vi "flow-builder.water-dosing.vi"(7 "Proc Name":string, 8 "error in":errorcluster, 9 "Unit Index":i32, 10 "AIN Simulator (NaN)":dbl=nan, 11 "Cluster":T3 {"ORP Dosing"."MIX Limit" format="%d [s]"; "ORP Dosing"."MIX Dose" format="%d [s]"; "PH Dosing"."ACID Limit" format="%d [s]"; "PH Dosing"."BASE Limit" format="%d [s]"; "PH Dosing"."ACID Dose" format="%d [s]"; "PH Dosing"."BASE Dose" format="%d [s]"; "EC Dosing"."BETA2 Limit" format="%d [s]"; "EC Dosing"."ALFA2 Limit" format="%d [s]"; "EC Dosing"."ALFA2 Dose" format="%d [s]"; "EC Dosing"."BETA2 Dose" format="%d [s]"; "EC Dosing"."BETA1 Limit" format="%d [s]"; "EC Dosing"."ALFA1 Limit" format="%d [s]"; "EC Dosing"."ALFA1 Dose" format="%d [s]"; "EC Dosing"."BETA1 Dose" format="%d [s]"; "Main"."DailyActivityHours"."Begin Time" format="ON:    %<%H:%M>T"; "Main"."DailyActivityHours"."End Time" format="OFF:    %<%H:%M>T"; "Main"."WashTimes"."Out" format="Wash out: %d [sec]"; "Main"."WashTimes"."In" format="Wash in: %d [sec]"; "Water Dosing"."Water Limit" format="%d [s]"; "Water Dosing"."Water Dose" format="%d [s]"}) -> (0 "error out":errorcluster, 1 "Not Limited?":bool, 2 "status":string, 3 "Flow out":T1[](array[typedef]))   [LabVIEW 2024]
uses:
  controls/UiNutritionPanel.ctl
  controls/UiScheduleTimestamp.ctl
  controls/UiStepBuilder.ctl
  controls/type.step-builder.ctl
  controls/enum-ntr-io-format.ctl
  io.interface.serial.vi
  <vilib>/Utility/error.llb/Clear Errors.vi
  Polymorphics/variantCtrlIo.vi
  globals/globals-engine.vi
  util.environment.vi
  util-address-parser.vi
  util-address-builder.vi
  util.DO.ToString.vi
  Polymorphics/io.command-builder.vi
  Polymorphics/io.command-builder.DO.vi
  Polymorphics/io.command-builder.AI.vi
  Polymorphics/io.command-builder.DI.vi
  io.frame.vi
  io.visa.vi
  io.responseValidator.vi
  Polymorphics/io.command-parser.DI.vi
  Polymorphics/io.command-parser.AI.vi
  step.util.flag-matching.vi
  util.file.record.vi
panel:
  # "Water"
  # "EC"
  # "PH"
  # "ORP"
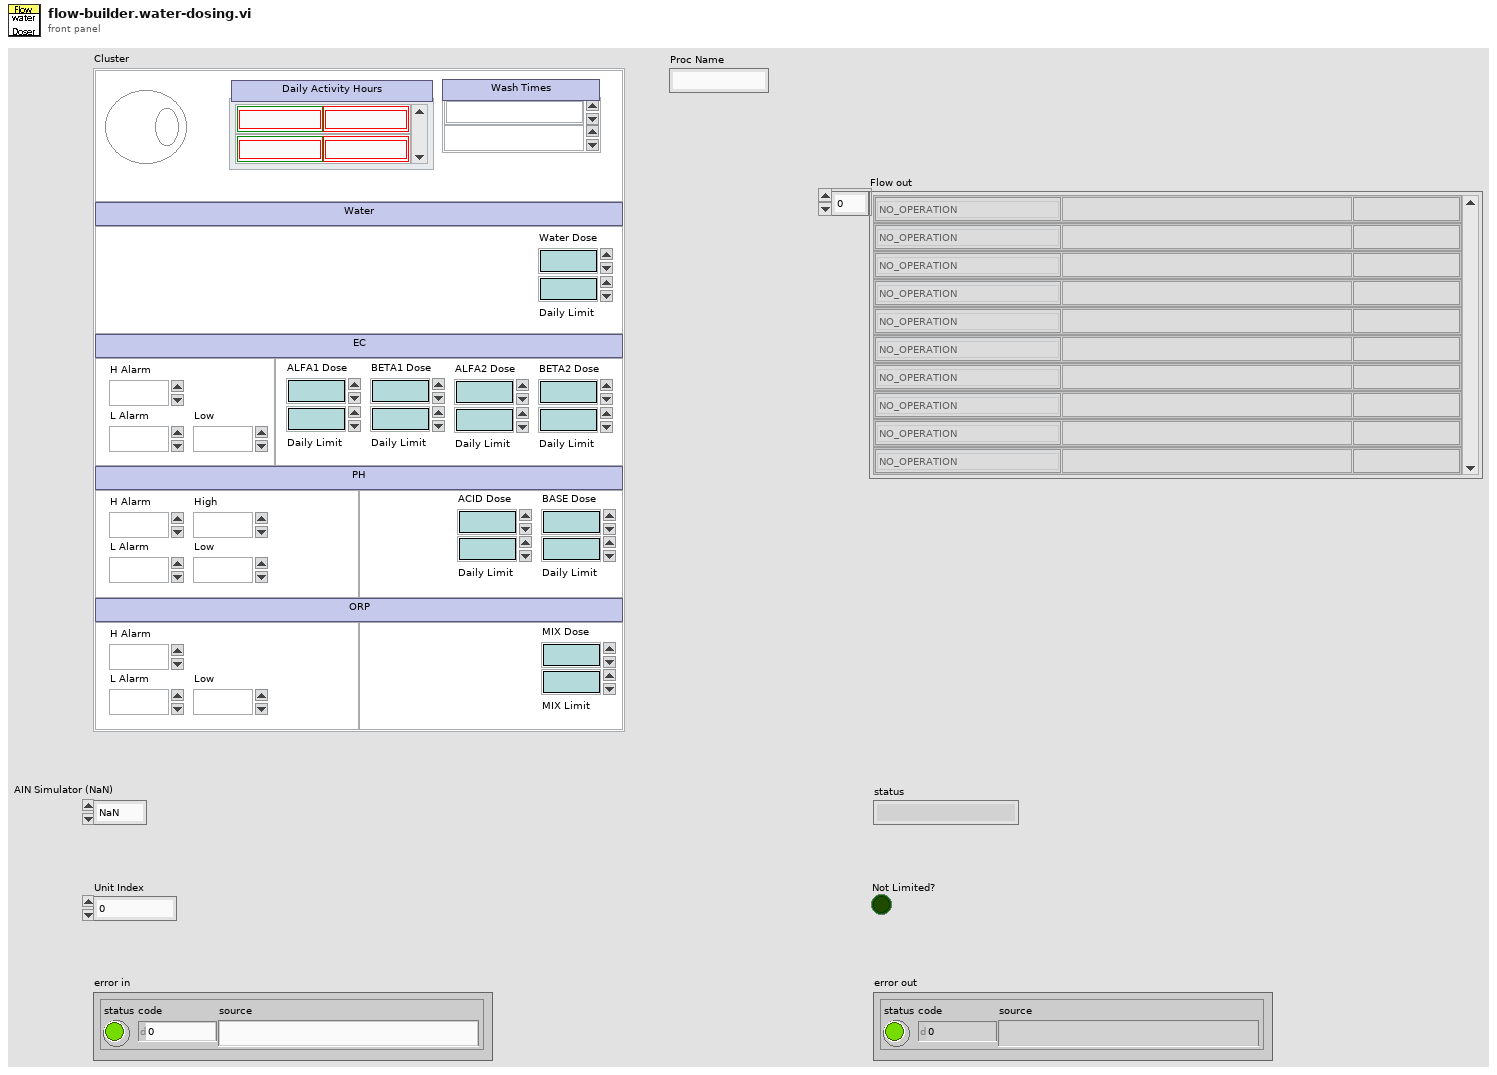
[diagram p1: front panel]
types:
  T1 = typedef "UiStepBuilder.ctl" = cluster{"Step Function":T2, "ParamString":string, "Step Label":string}
  T2 = typedef "type.step-builder.ctl" = enum16{"NO_OPERATION", "DELAY-JUMP", "DELAY", "JUMP", "COMPLETE", "SCHEDULER", "IRR-CHECK", "UNIT-CHECK", "UNIT-SAMPLE", "UNIT-DOSE", "LOG-REPORT", "LOG-MESSAGE", "IO-READ", "IO-READ-MANY", "IO-WRITE", "IO-COMPARE-OUT", "IO-COMPARE-IN", "PROC-START", "PROC-STOP", "PROC-LOAD", "PROC-IS-COMPLETED", "RECORD-MOVE", "GET-RH", "GET-UV", "GET-WD", "GET-WS", "OCS-CHECK", "OCS-RECORD"}
  T3 = typedef "UiNutritionPanel.ctl" = cluster{"Main":cluster{"Enable":bool, "WashTimes":cluster{"In":dbl, "Out":dbl}, "DailyActivityHours":cluster{"Begin Time":T4, "End Time":T4}[]}, "Water Dosing":cluster{"Water Dose":dbl, "Water Limit":dbl}, "EC Ranges":cluster{"H Alarm":dbl, "L Alarm":dbl, "Low":dbl}, "EC Dosing":cluster{"ALFA1 Dose":dbl, "ALFA1 Limit":dbl, "BETA1 Dose":dbl, "BETA1 Limit":dbl, "ALFA2 Dose":dbl, "ALFA2 Limit":dbl, "BETA2 Dose":dbl, "BETA2 Limit":dbl}, "PH Ranges":cluster{"H Alarm":dbl, "L Alarm":dbl, "High":dbl, "Low":dbl}, "PH Dosing":cluster{"ACID Dose":dbl, "ACID Limit":dbl, "BASE Dose":dbl, "BASE Limit":dbl}, "ORP Ranges":cluster{"H Alarm":dbl, "L Alarm":dbl, "Low":dbl}, "ORP Dosing":cluster{"MIX Dose":dbl, "MIX Limit":dbl}}
  T4 = typedef "UiScheduleTimestamp.ctl" = timestamp
  T5 = typedef "enum-ntr-io-format.ctl" = enum16{"UN_VLV%d", "UN_PMP%d", "UN_WL%d", "UN_PH", "UN_EC", "UN_ORP", "UN_WT", "UN_PH2", "UN_ALFA1", "UN_BETA1", "UN_ALFA2", "UN_BETA2", "UN_ACID", "UN_BASE", "UN_WATER", "UN_ORPMIX"}
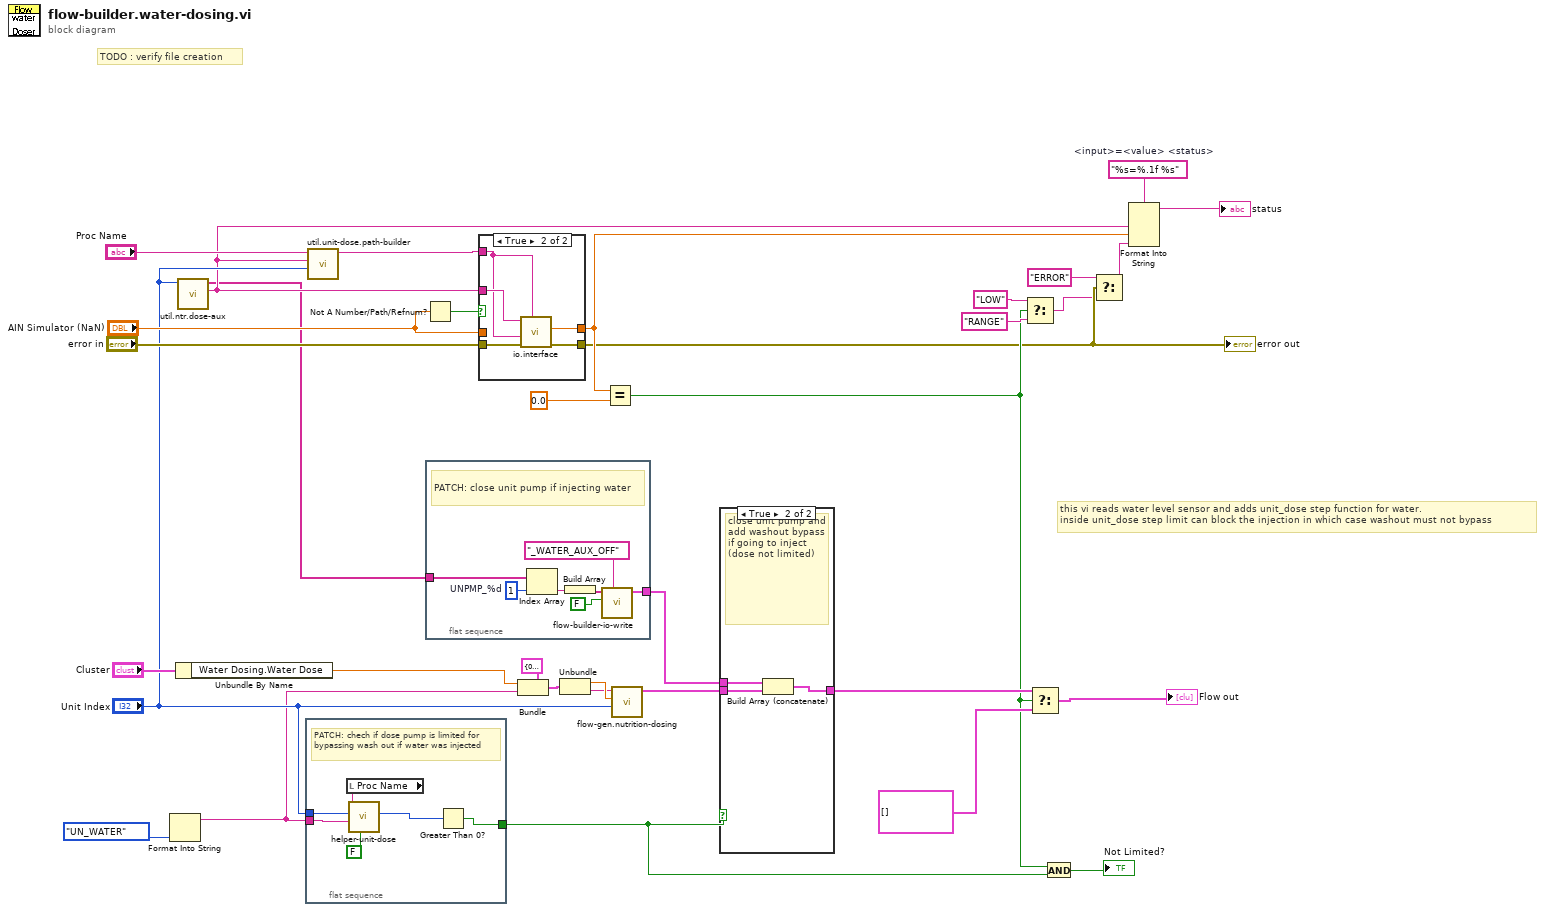
[diagram p0: block diagram]
diagram:
  w31 = "%s=%.1f %s"  # <input>=<value> <status>
  # "TODO : verify file creation"
  # "this vi reads water level sensor and adds unit_dose step function for water.\ninside unit_dose step limit can block the injection in which case washout must not bypass"
  n1 = Format Into String(enum-ntr-io-format."UN_WATER") -> (resulting string=w1:string)  [unwired: 3 in, 1 out]
  n2 = Unbundle By Name("Cluster") -> ("Water Dosing.Water Dose"=w27:dbl)
  n3 = call "util.ntr.dose-aux.vi"("Unit Index"="Unit Index") -> ("Unit Water Level (UN_WL%d)"=w8:string, "DO Unit Pumps"=w7:string[])  [unwired: 6 in, 3 out]
  n4 = flat-sequence {
    tunnel: "Unit Index" -> [w39]
    tunnel: w1 -> [w38]
    tunnel: [w36] -> w19
    frame #0 {
      # "PATCH: chech if dose pump is limited for bypassing wash out if water was injected"
      n5 = local read "Proc Name"() -> (w40:string)
      n6 = call "helper-unit-dose.vi"("Auto Update Limit Record? (T)"=FALSE ("(F)ReadOnly/(T)Auto Update"), "output"=w38, "Unit Index"=w39, "Proc Name"=w40) -> ("Actual Dose in Seconds"=w37:i32)  [unwired: 5 in, 2 out]
      n7 = Greater Than 0?(x=w37) -> (x > 0?=w36:bool)
    }
  }
  n8 = call "util.unit-dose.path-builder.vi"("Unit Index"="Unit Index", "Input"=w8, "Proc Name"="Proc Name") -> ("\\NUTRITION\\ORP\\ORP_U1_2024-08-16.*"=w11:string)  [unwired: 8 in]
  n9 = Not A Number/Path/Refnum?(number/path/refnum="AIN Simulator (NaN)") -> (NaN/Path/Refnum?=w14:bool)
  n10 = flat-sequence {
    tunnel: [w46] -> w18
    tunnel: w7 -> [w44]
    frame #0 {
      w45 = 1  # UNPMP_%d
      # "PATCH: close unit pump if injecting water"
      n11 = Index Array(array=w44, index=w45) -> (element=w43:string)
      n12 = Build Array(w43) -> (w42:string[])
      n13 = call "flow-builder-io-write.vi"("Step Name"="_WATER_AUX_OFF" ("format string"), "Value in"=FALSE, "Dout+AUX"=w42) -> ("Flow out"=w46:T1[])  [unwired: 8 in]
    }
  }
  n14 = case shown="True" w14 {
    tunnel: w8 -> [_ w54]
    tunnel: [w49 w53] -> w30
    tunnel: [w48 w52] -> w5
    tunnel: "error in" -> [w48 w51]
    tunnel: "AIN Simulator (NaN)" -> [w49 _]
    tunnel: w11 -> [_ w50]
    frame False {
    }
    frame True {
      n15 = call "io.interface.vi"("Caller"=w50, "error in"=w51, "record filename.* (disabled if empty)"=w50, "IO Name in"=w54) -> ("error out"=w52:errorcluster, "Value out"=w53:dbl)  [unwired: 2 in, 4 out]
    }
  }
  "error out" <- w5
  n16 = Bundle(cluster=cluster{"Dose Time":dbl, "Input":string} {"Dose Time"=0.0, "Input"=""} ("Cluster"), "Dose Time"=w27, "Input"=w1) -> (w21:cluster{"Dose Time":dbl, "Input":string})
  n17 = Unbundle(w21) -> ("Dose Time"=w23:dbl, "Input"=w22:string)
  n18 = Equal?(x=w30, y=0.0) -> (x = y?=w16:bool)
  n19 = call "flow-gen.nutrition-dosing.vi"("Unit Index"="Unit Index", "Dosing Time"=w23, "IO Name"=w22) -> ("Flow"=w25:T1[])  [unwired: 7 in, 1 out]
  n20 = case shown="True" w19 {
    tunnel: w25 -> [w55 w58]
    tunnel: [w55 w57] -> w24
    tunnel: w18 -> [_ w56]
    frame False {
      # "dose punp is limit, go to dose pump step (to generate limit log) but w/o  closing aux pump"
    }
    frame True {
      # "close unit pump and add washout bypass if going to inject (dose not limited)"
      n21 = Build Array (concatenate)(w56, w58) -> (w57:T1[])
    }
  }
  n22 = Select(t="LOW", s=w16, f="RANGE") -> (s? t:f=w4:string)
  n23 = Select(t=w24, s=w16, f=T1[] []) -> (s? t:f=→"Flow out":T1[])
  n24 = And(x=w16, y=w19) -> (x .and. y?=→"Not Limited?":bool)
  n25 = Select(t="ERROR", s=w5, f=w4) -> (s? t:f=w3:string)
  n26 = Format Into String(format string=w31, w8, w30, w3) -> (resulting string=→"status":string)  [unwired: 2 in, 1 out]
